vi "GET_AllData.vi"(8 "error in (no error)":errorcluster, 11 "FakedArray.lvclass in":refnum<class "FakedArray.lvclass">) -> (0 "error out":errorcluster, 2 "Data":variant, 3 "FakedArray.lvclass out":refnum<class "FakedArray.lvclass">)   [LabVIEW 2021, in "FakedArray.lvclass"]
uses:
  <resource>/plugins/NIIconEditor/Class/FakedArray/FakedArray.lvclass
  <resource>/plugins/NIIconEditor/Class/FakedArray/FakedArray.lvclass/FakedArray.ctl
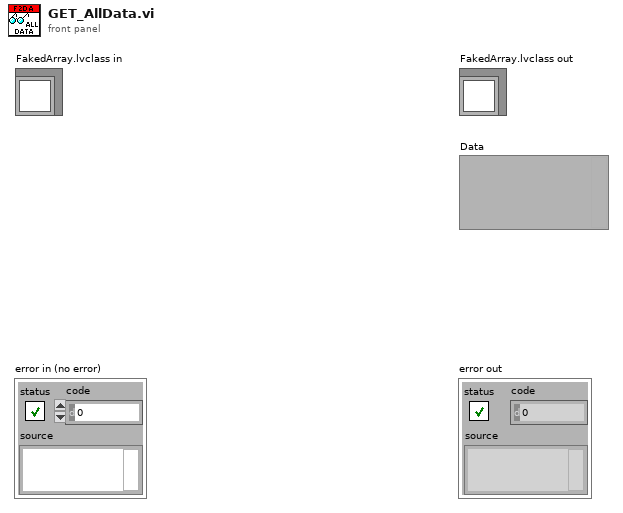
[diagram p1: front panel]
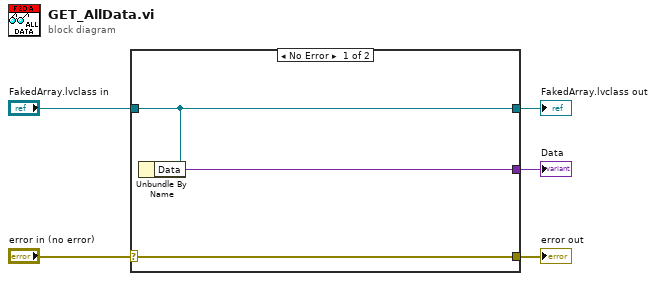
[diagram p0: block diagram]
diagram:
  n1 = case shown="No Error" "error in (no error)" {
    selector: "error in (no error)" -> [w8 w9]
    tunnel: [w8 w9] -> w4
    tunnel: [w7 w10] -> w2
    tunnel: "FakedArray.lvclass in" -> [w7 w10]
    tunnel: [w6 _] -> w1
    frame No Error {
      n2 = Unbundle By Name(w7) -> ("Data"=w6:variant)
    }
    frame Error {
    }
  }
  "error out" <- w4
  "FakedArray.lvclass out" <- w2
  "Data" <- w1
